vi "Basic Linked List Test.vi"() -> ()   [LabVIEW 2019]
uses:
  <vilib>/gpm_packages/@cs/linked-list/Source/Linked List/Linked List/Linked List.lvclass
  C:/Program Files/National Instruments/LabVIEW 2019/vi.lib/gpm_packages/@cs/linked-list/Source/Linked List/ILinkedList/ILinked List.lvclass
  <vilib>/gpm_packages/@cs/persistence/source/XML/XML.lvclass
  C:/Program Files/National Instruments/LabVIEW 2019/vi.lib/gpm_packages/@cs/persistence/source/IPersist/IPersist.lvclass
  ccde8f49-4a17-49cc-9737-dcb58406fc16.vi
  dab86994-a063-497e-9468-bd44bcc8ce0e.vi
  b58670ae-db1f-4200-b1b0-b8ca0885bd08.vi
  b4c9c6a9-1723-4f72-87fd-a7ed9d973242.vi
  44534c4a-a207-4f38-9c96-8b042e4336ab.vi
  338610e7-be63-416b-893d-33345bc18be6.vi
  aa432d14-afcb-44d9-84f6-5287c3fb00b2.vi
  7b3718cf-712b-4f78-ad0f-875d7a3644d5.vi
  89ea6514-41bc-4baf-997a-08f19e4a663b.vi
  2995618f-ceea-45ce-8b0f-beb3f7c83228.vi
  8995b677-d4a3-45ec-ac8a-8d1396ff8e75.vi
  f624bd61-55be-46eb-abf3-2dcedbbdb1dc.vi
  d4a9b6b4-3b48-4807-aa76-34d27f98f90f.vi
  <vilib>/Utility/error.llb/Clear Errors.vi
  <vilib>/gpm_packages/@cs/linked-list/Source/Linked List/ILinkedList/ILinked List.lvclass
  <vilib>/gpm_packages/@cs/linked-list/Source/Linked List/Linked List Ref/Linked List Ref.lvclass
panel:
  out "Attribute":i32
  out "Data ID 4":string
  out "Age":i32
  out "Data ID 3":string
  out "Attribute 5":i32
  out "Attribute 4":i32
  out "Attribute 3":i32
  out "Attributes":i32[](array[numeric])
  in  "Tree 3":string(tree)
  out "Data ID 2":string
  out "Data ID":string
  out "Names":string[](array[string])
  out "IDs":string[](array[string])
  out "Attribute ID out":string
  in  "Tree 2":string(tree)
  in  "Tree":string(tree)
  out "Found?":bool
  out "Attribute 2":i32
  out "Attribute Name out 2":string
  in  "File Name":string
  in  "Folder":path
  out "error out":errorcluster
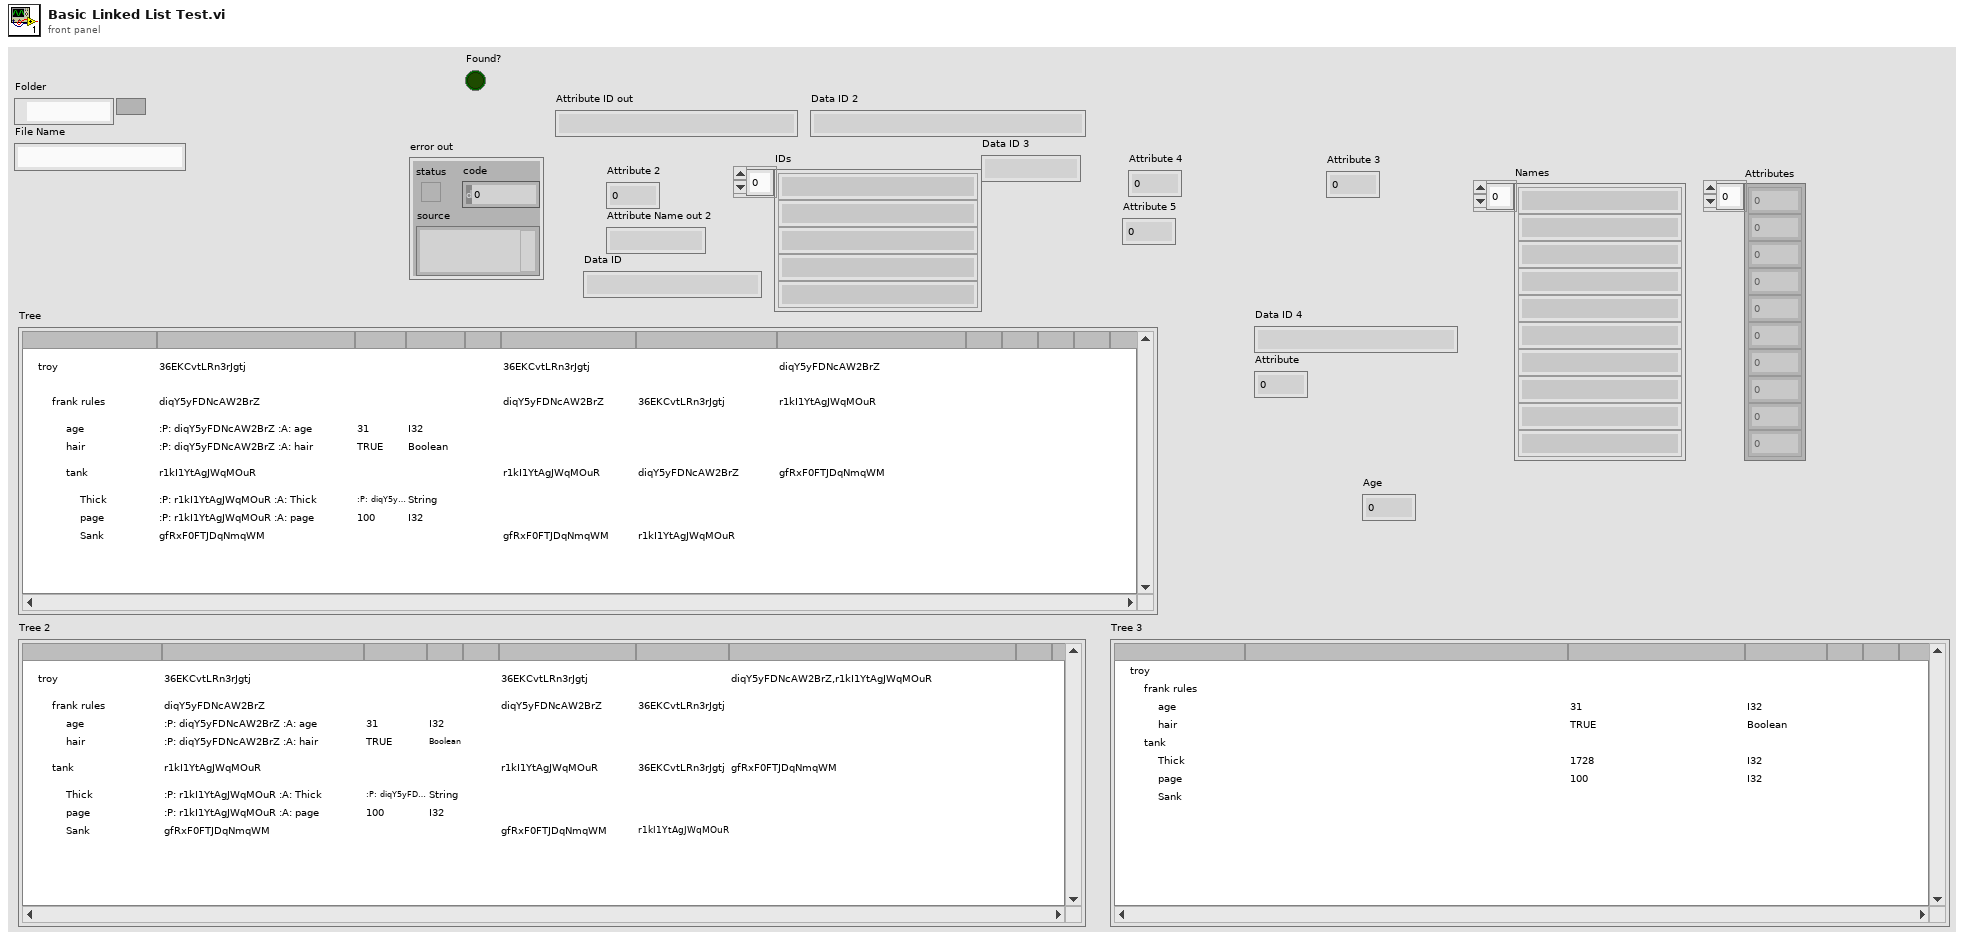
[diagram p1: front panel]
types:
  T1 = cluster{"Left Cell String":string, "Child Text":string[], "Child Tag":string, "Item Indent":i32, "Child Only?":bool, "Glyph Index":i32}[]
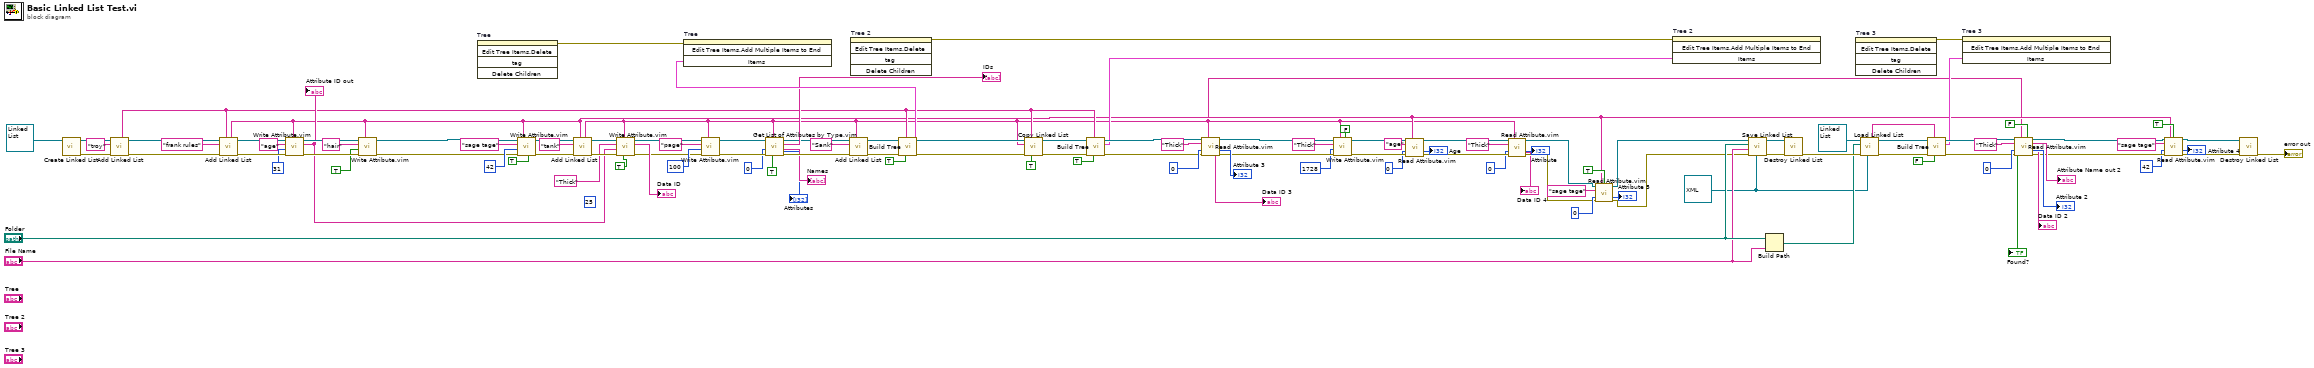
[diagram p0: block diagram]
diagram:
  (unwired) 25
  w60 = refnum<class "XML.lvclass"> refnum ("Dictionary.lvlib:XML.lvclass")
  n1 = call <vilib>:"Create Linked List.vi"("Linked List"=refnum<class "Linked List.lvclass"> refnum ("Dictionary.lvlib:Dictionary.lvclass")) -> ("error out"=w95:errorcluster, "Linked List Ref"=w97:refnum<data-value>)  [unwired: 9 in]
  n2 = call <vilib>:"Add Linked List.vi"("error in (no error)"=w95, "Name"="troy" ("Dictionary Name"), "Linked List Ref"=w97) -> ("error out"=w94:errorcluster, "Linked List Ref out"=w96:refnum<data-value>, "Linked List ID out"=w43:string)  [unwired: 5 in, 1 out]
  n3 = call <vilib>:"Add Linked List.vi"("Parent ID"=w43, "error in (no error)"=w94, "Name"="frank rules", "Linked List Ref"=w96) -> ("error out"=w118:errorcluster, "Linked List Ref out"=w119:refnum<data-value>, "Linked List ID out"=w14:string)  [unwired: 4 in, 1 out]
  n4 = call "Write Attribute.vim"("Linked List ID"=w14, "error in (no error)"=w118, "Attribute"=31, "Attribute Name"="age", "Linked List Ref"=w119) -> ("error out"=w114:errorcluster, "Attribute ID out"=w86:string, "Linked List Ref out"=w115:refnum<data-value>)  [unwired: 3 in, 1 out]
  "Attribute ID out" <- w86
  n5 = call "Write Attribute.vim"("Linked List ID"=w14, "error in (no error)"=w114, "Attribute"=TRUE, "Attribute Name"="hair", "Linked List Ref"=w115) -> ("error out"=w34:errorcluster, "Linked List Ref out"=w35:refnum<data-value>)  [unwired: 3 in, 2 out]
  n6 = invoke on="Tree" class="Tree (strict)" method="Edit Tree Items.Delete"() -> (error out=w103:errorcluster)  [unwired: 5 in, 4 out]
  n7 = call "Write Attribute.vim"("Private?"=TRUE, "Linked List ID"=w14, "error in (no error)"=w34, "Attribute"=42, "Attribute Name"="sage tage", "Linked List Ref"=w35) -> ("error out"=w76:errorcluster, "Linked List Ref out"=w77:refnum<data-value>)  [unwired: 2 in, 2 out]
  n8 = call <vilib>:"Add Linked List.vi"("Parent ID"=w14, "error in (no error)"=w76, "Name"="tank", "Linked List Ref"=w77) -> ("error out"=w90:errorcluster, "Linked List Ref out"=w91:refnum<data-value>, "Linked List ID out"=w10:string)  [unwired: 4 in, 1 out]
  n9 = call "Write Attribute.vim"("Pointer?"=TRUE, "Linked List ID"=w10, "error in (no error)"=w90, "Attribute"=w86, "Attribute Name"="Thick", "Linked List Ref"=w91) -> ("error out"=w70:errorcluster, "Attribute ID out"=→"Data ID":string, "Linked List Ref out"=w71:refnum<data-value>)  [unwired: 2 in, 1 out]
  n10 = call "Write Attribute.vim"("Linked List ID"=w10, "error in (no error)"=w70, "Attribute"=100, "Attribute Name"="page", "Linked List Ref"=w71) -> ("error out"=w54:errorcluster, "Linked List Ref out"=w55:refnum<data-value>)  [unwired: 3 in, 2 out]
  n11 = call "Get List of Attributes by Type.vim"("Recurse Up List (Default=True)"=TRUE, "Linked List ID"=w10, "error in (no error)"=w54, "Type"=0, "Linked List Ref"=w55) -> ("error out"=w57:errorcluster, "Names"=→"Names":string[], "IDs"=→"IDs":string[], "Linked List Ref out"=w58:refnum<data-value>, "Attributes"=→"Attributes":i32[])  [unwired: 2 in]
  n12 = call <vilib>:"Add Linked List.vi"("Parent ID"=w10, "error in (no error)"=w57, "Name"="Sank", "Linked List Ref"=w58) -> ("error out"=w45:errorcluster, "Linked List Ref out"=w47:refnum<data-value>)  [unwired: 4 in, 2 out]
  n13 = invoke on="Tree 2" class="Tree (strict)" method="Edit Tree Items.Delete"() -> (error out=w100:errorcluster)  [unwired: 5 in, 4 out]
  n14 = call <vilib>:"Build Tree.vi"("Show IDs"=TRUE, "Linked List ID"=w43, "error in (no error)"=w45, "Linked List Ref"=w47) -> ("error out"=w44:errorcluster, "Tree Data"=w102:T1, "Linked List Ref out"=w46:refnum<data-value>)  [unwired: 5 in]
  n15 = invoke on="Tree" class="Tree (strict)" method="Edit Tree Items.Add Multiple Items to End"(error in=w103, "Items"=w102) -> ()  [unwired: 2 in, 4 out]
  n16 = call <vilib>:"Copy Linked List.vi"("Move?"=TRUE, "New Parent Linked List ID"=w43, "error in (no error)"=w44, "Linked List ID"=w10, "Linked List Ref"=w46) -> ("error out"=w50:errorcluster, "Linked List Ref out"=w52:refnum<data-value>)  [unwired: 3 in, 2 out]
  n17 = call <vilib>:"Build Tree.vi"("Show IDs"=TRUE, "Linked List ID"=w43, "error in (no error)"=w50, "Linked List Ref"=w52) -> ("error out"=w49:errorcluster, "Tree Data"=w48:T1, "Linked List Ref out"=w51:refnum<data-value>)  [unwired: 5 in]
  n18 = call "Read Attribute.vim"("Linked List Ref"=w51, "Linked List ID"=w10, "Attribute Name"="Thick", "Type"=0, "error in (no error)"=w49) -> ("Linked List Ref out"=w20:refnum<data-value>, "Attribute"=→"Attribute 3":i32, "Data ID"=→"Data ID 3":string, "error out"=w19:errorcluster)  [unwired: 5 in, 2 out]
  n19 = call "Write Attribute.vim"("Update Pointer?"=FALSE, "Linked List ID"=w10, "error in (no error)"=w19, "Attribute"=1728, "Attribute Name"="Thick", "Linked List Ref"=w20) -> ("error out"=w15:errorcluster, "Linked List Ref out"=w16:refnum<data-value>)  [unwired: 2 in, 2 out]
  n20 = call "Read Attribute.vim"("Linked List Ref"=w16, "Linked List ID"=w14, "Attribute Name"="age", "Type"=0, "error in (no error)"=w15) -> ("Linked List Ref out"=w9:refnum<data-value>, "Attribute"=→"Age":i32, "error out"=w6:errorcluster)  [unwired: 5 in, 3 out]
  n21 = call "Read Attribute.vim"("Linked List Ref"=w9, "Linked List ID"=w10, "Attribute Name"="Thick", "Type"=0, "error in (no error)"=w6) -> ("Linked List Ref out"=w8:refnum<data-value>, "Attribute"=→"Attribute":i32, "Data ID"=→"Data ID 4":string, "error out"=w5:errorcluster)  [unwired: 5 in, 2 out]
  n22 = call "Read Attribute.vim"("Linked List Ref"=w8, "Linked List ID"=w14, "Include Private?"=TRUE, "Attribute Name"="sage tage", "Type"=0, "error in (no error)"=w5) -> ("Linked List Ref out"=w37:refnum<data-value>, "Attribute"=→"Attribute 5":i32, "error out"=w36:errorcluster)  [unwired: 4 in, 3 out]
  n23 = invoke on="Tree 2" class="Tree (strict)" method="Edit Tree Items.Add Multiple Items to End"(error in=w100, "Items"=w48) -> ()  [unwired: 2 in, 4 out]
  n24 = call <vilib>:"Save Linked List.vi"("Persistence"=w60, "error in (no error)"=w36, "File Name"="File Name", "Folder"="Folder", "Linked List Ref"=w37) -> ("error out"=w84:errorcluster, "Linked List Ref out"=w85:refnum<data-value>)  [unwired: 5 in]
  n25 = Build Path(base path="Folder", name or relative path="File Name") -> (appended path=w110:path)
  n26 = call <vilib>:"Destroy Linked List.vi"("error in (no error)"=w84, "Linked List Ref"=w85) -> ("error out"=w111:errorcluster)  [unwired: 9 in]
  n27 = invoke on="Tree 3" class="Tree (strict)" method="Edit Tree Items.Delete"() -> (error out=w80:errorcluster)  [unwired: 5 in, 4 out]
  n28 = call <vilib>:"Load Linked List.vi"("Persistence"=w60, "error in (no error)"=w111, "File Path"=w110, "Linked List"=refnum<class "Linked List.lvclass"> refnum ("Dictionary.lvlib:Dictionary.lvclass")) -> ("error out"=w64:errorcluster, "Linked List Ref out"=w65:refnum<data-value>, "Linked List ID out"=w63:string)  [unwired: 5 in]
  n29 = call <vilib>:"Build Tree.vi"("Show IDs"=FALSE, "Linked List ID"=w63, "error in (no error)"=w64, "Linked List Ref"=w65) -> ("error out"=w82:errorcluster, "Tree Data"=w79:T1, "Linked List Ref out"=w83:refnum<data-value>)  [unwired: 5 in]
  n30 = invoke on="Tree 3" class="Tree (strict)" method="Edit Tree Items.Add Multiple Items to End"(error in=w80, "Items"=w79) -> ()  [unwired: 2 in, 4 out]
  n31 = call "Read Attribute.vim"("Linked List Ref"=w83, "Linked List ID"=w10, "Flatten Pointer?"=FALSE, "Attribute Name"="Thick", "Type"=0, "error in (no error)"=w82) -> ("Linked List Ref out"=w41:refnum<data-value>, "Attribute Name out"=→"Attribute Name out 2":string, "Attribute"=→"Attribute 2":i32, "Found?"=→"Found?":bool, "Data ID"=→"Data ID 2":string, "error out"=w39:errorcluster)  [unwired: 4 in]
  n32 = call "Read Attribute.vim"("Linked List Ref"=w41, "Linked List ID"=w14, "Include Private?"=TRUE, "Attribute Name"="sage tage", "Type"=42, "error in (no error)"=w39) -> ("Linked List Ref out"=w40:refnum<data-value>, "Attribute"=→"Attribute 4":i32, "error out"=w38:errorcluster)  [unwired: 4 in, 3 out]
  n33 = call <vilib>:"Destroy Linked List.vi"("error in (no error)"=w38, "Linked List Ref"=w40) -> ("error out"=→"error out":errorcluster)  [unwired: 9 in]
